vi "Peak Detection sub.vi"(9 "peak number":i32, 11 "tirgger signal":dbl[](array[numeric]) format="%0.3f") -> (1 "x value of peak":dbl, 3 "Count of Peaks":i32)   [LabVIEW 2014]
uses:
  <vilib>/Analysis/NI_AAL_SigProc.lvlib
panel:
  out "Peaks on Trigger":T1(graph)
  out "Trigger Signal":dbl[](graph)
  out "Differentiated Signal":dbl[](graph)
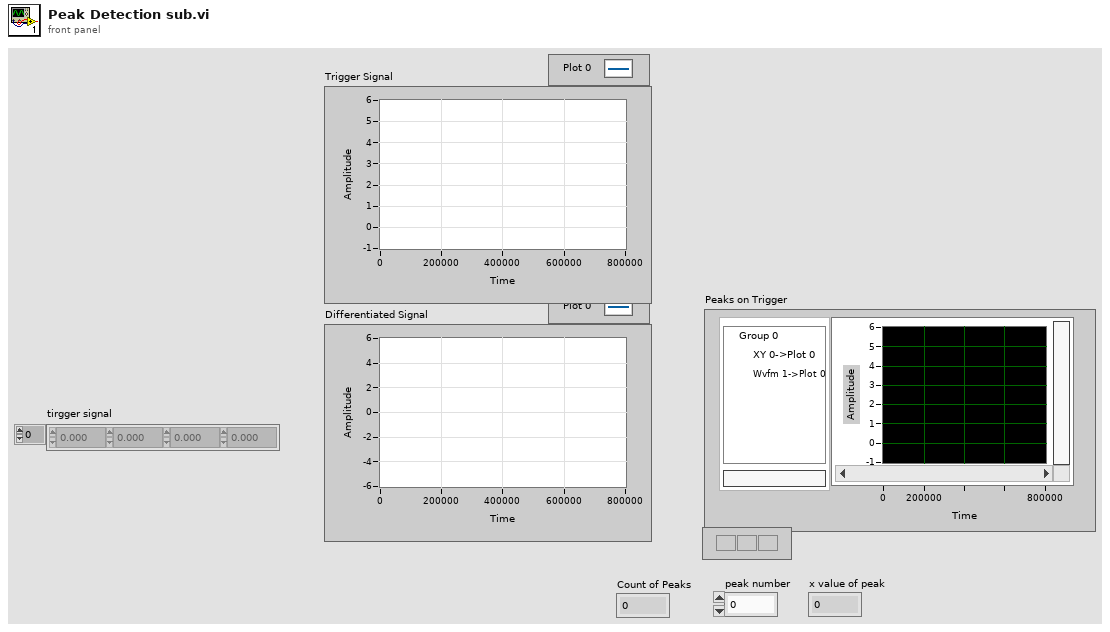
[diagram p1: front panel]
types:
  T1 = cluster{cluster{dbl[], "Amplitudes":dbl[]}, waveform(dbl)}
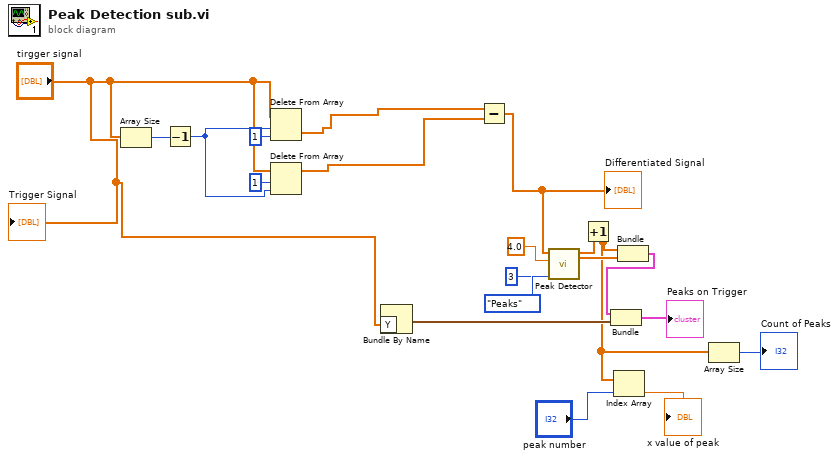
[diagram p0: block diagram]
diagram:
  n1 = Array Size(array="tirgger signal") -> (size(s)=w10:i32)
  n2 = Decrement(x=w10) -> (x-1=w18:i32)
  n3 = Delete From Array(array="tirgger signal", length=w18, index=1) -> (deleted portion=w17:dbl[])  [unwired: 1 out]
  n4 = Delete From Array(array="tirgger signal", length=1, index=w18) -> (array with subset deleted=w16:dbl[])  [unwired: 1 out]
  n5 = Bundle By Name("Y"="tirgger signal") -> (w8:waveform(dbl))  [unwired: 1 in]
  n6 = Subtract(x=w17, y=w16) -> (x-y=w5:dbl[])
  "Differentiated Signal" <- w5
  n7 = call <vilib>:"Peak Detector.vi"("peaks/valleys"=enum32{"Peaks", "Valleys"}."Peaks", "width"=3, "threshold"=4.0, "X"=w5) -> ("Amplitudes"=w12:dbl[], "Locations"=w11:dbl[])  [unwired: 3 in, 3 out]
  n8 = Increment(x=w11) -> (x+1=w2:dbl[])
  n9 = Index Array(array=w2, index="peak number") -> (element=→"x value of peak":dbl)
  n10 = Bundle(w2, "Amplitudes"=w12) -> (w9:cluster{dbl[], "Amplitudes":dbl[]})  [unwired: 1 in]
  n11 = Bundle(w9, w8) -> (→"Peaks on Trigger":T1)  [unwired: 1 in]
  n12 = Array Size(array=w2) -> (size(s)=→"Count of Peaks":i32)
  "Trigger Signal" <- "tirgger signal"
